vi "Application Name--constant.vi"() -> (3 "Application Name":string="HV-60D Application v1.0")   [LabVIEW 2018, in "Application.lvlib"]
doc: "Return the Application name.\n_____\nBased on DQMH Project Template 6.0.0.91."
uses:
  Application.lvlib
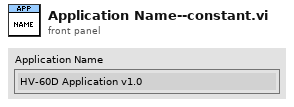
[diagram p1: front panel]
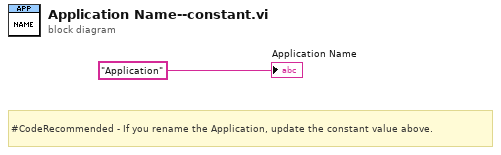
[diagram p0: block diagram]
diagram:
  # "#CodeRecommended - If you rename the Application, update the constant value above."
  "Application Name" <- "Application" ("Application Name 2")
